vi "Compile Analog Replay 1.0 Data.vi"(7 "RIO Address":string, 8 "error in (no error)":errorcluster, 11 "Device Item Ref in":T3 format="%.0x") -> (0 "error out":errorcluster, 1 "bitfile names":string[](array[string]), 2 "Analog Replays":T1[](array[typedef]), 3 "Device Item Ref out":T3 format="%.0x")   [LabVIEW 2019, in "Engine Simulation Toolkit System Explorer.lvlib"]
uses:
  Engine Simulation Toolkit System Explorer.lvlib
  <vilib>/NI VeriStand/Custom Device API/Custom Device Item Ref.ctl
  Shared/1.0 Analog Replay Engine Data.ctl
  Shared/1.0 Analog Replay FIFO Idxs.ctl
  Position Reference.ctl
  Shared/Properties.vi
  Shared/Constants and GUIDs.vi
  <vilib>/NI VeriStand/Custom Device Tools/Custom Device Utility Library/NI VeriStand - Search for Item by GUID.vi
  <vilib>/NI VeriStand/Custom Device API/Get Item Property (String).vi
  <vilib>/NI VeriStand/Custom Device API/Get Item Property (Boolean).vi
  <vilib>/NI VeriStand/Custom Device API/Get Item Property (U16).vi
  <vilib>/NI VeriStand/Custom Device API/Get Item Property (Double).vi
  Shared/Engine Simulation Toolkit Shared.lvlib
  <vilib>/NI VeriStand/Custom Device API/Custom Device API.lvlib
  <vilib>/NI VeriStand/Custom Device Tools/Custom Device Utility Library/Custom Device Utility Library.lvlib
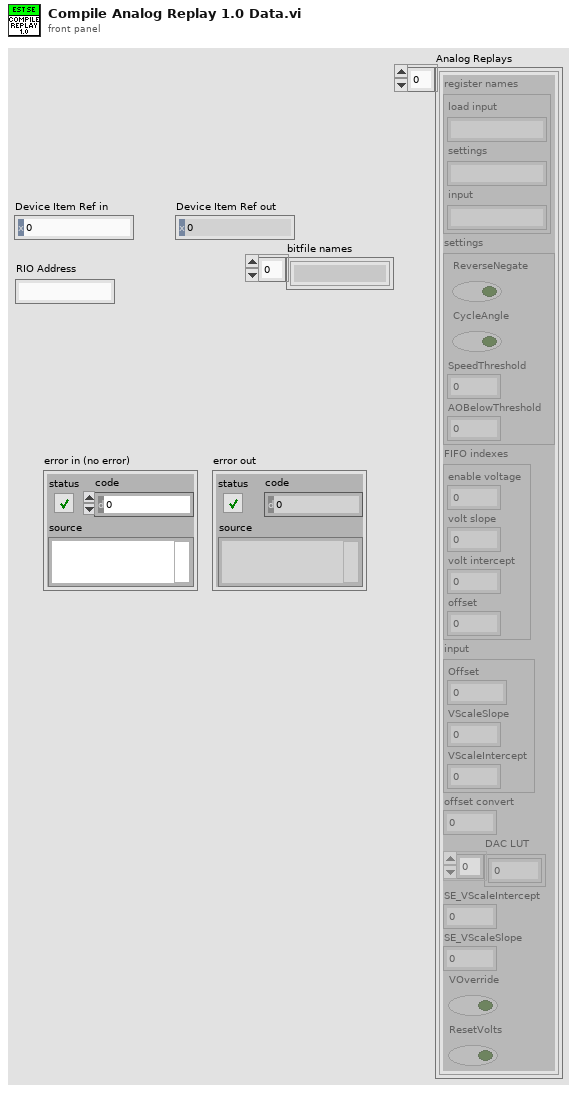
[diagram p1: front panel]
types:
  T1 = typedef "Engine Simulation Toolkit Shared.lvlib/1.0 Analog Replay Engine Data.ctl" = cluster{"register names":cluster{"load input":string, "settings":string, "input":string}, "settings":cluster{"ReverseNegate":bool, "CycleAngle":bool, "SpeedThreshold":fxp<+/-,23,2>, "AOBelowThreshold":i16}, "FIFO indexes":T2, "input":cluster{"Offset":i16, "VScaleSlope":fxp<+,18,6>, "VScaleIntercept":fxp<+/-,18,3>}, "offset convert":dbl, "DAC LUT":i16[], "SE_VScaleIntercept":fxp<+/-,18,3>, "SE_VScaleSlope":fxp<+,18,6>, "VOverride":bool, "ResetVolts":bool}
  T2 = typedef "Engine Simulation Toolkit Shared.lvlib/1.0 Analog Replay FIFO Idxs.ctl" = cluster{"enable voltage":i32, "volt slope":i32, "volt intercept":i32, "offset":i32}
  T3 = typedef "Custom Device API.lvlib/Custom Device Item Ref.ctl" = u64
  T4 = typedef "Engine Simulation Toolkit System Explorer.lvlib/Position Reference.ctl" = enum16{"Crank angle", "Cycle angle"}
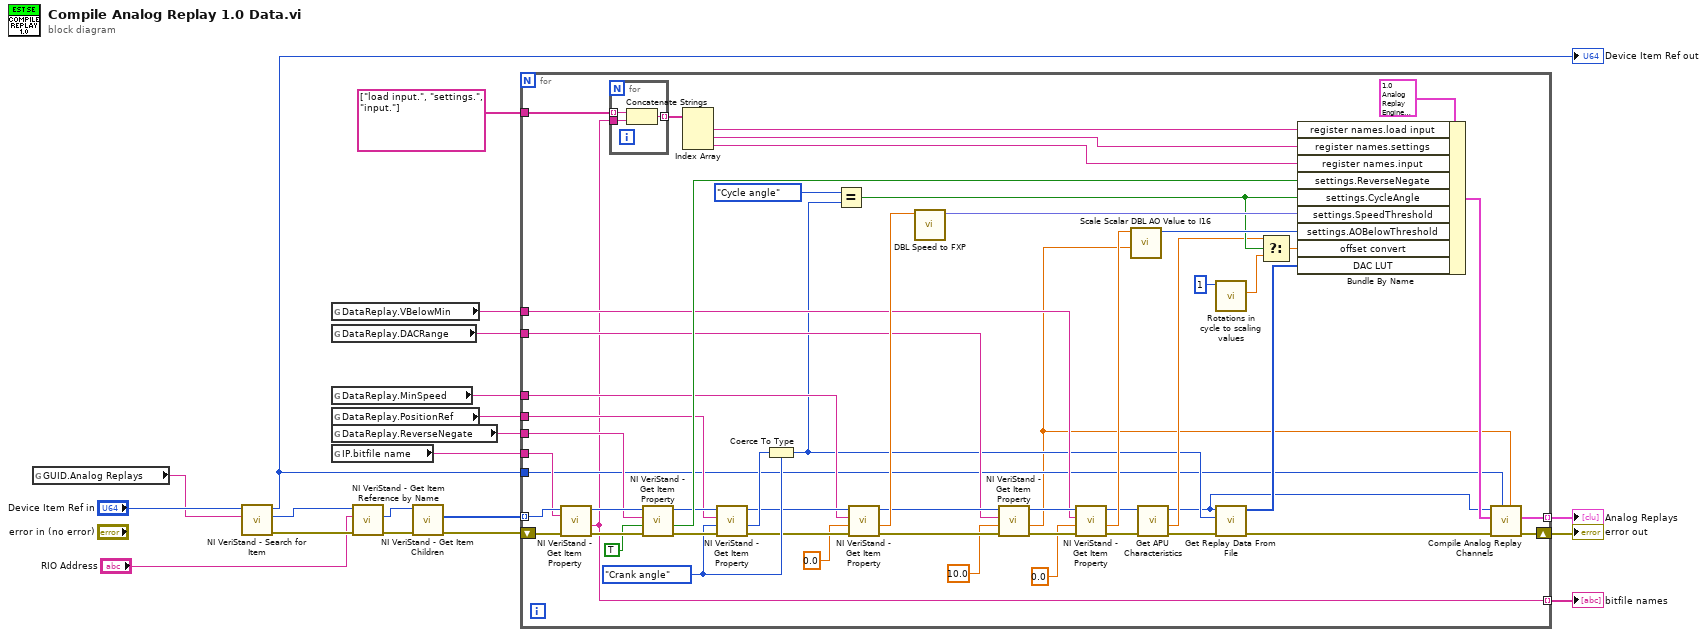
[diagram p0: block diagram]
diagram:
  n1 = global read "Constants and GUIDs.vi" "GUID.Analog Replays"() -> (w7:string)
  n2 = call-poly <vilib>:"NI VeriStand - Search for Item.vi"("Item GUID"=w7, "Section Ref in"="Device Item Ref in") -> ("error out"=w3:errorcluster, "Item Ref"=w6:T3, "Section Ref out"=w1:T3)  [unwired: 6 in, 1 out]
  "Device Item Ref out" <- w1
  n3 = global read "Properties.vi" "DataReplay.VBelowMin"() -> (w11:string)
  n4 = global read "Properties.vi" "DataReplay.DACRange"() -> (w12:string)
  n5 = global read "Properties.vi" "DataReplay.MinSpeed"() -> (w14:string)
  n6 = global read "Properties.vi" "DataReplay.PositionRef"() -> (w15:string)
  n7 = global read "Properties.vi" "DataReplay.ReverseNegate"() -> (w17:string)
  n8 = global read "Properties.vi" "IP.bitfile name"() -> (w19:string)
  n9 = call <vilib>:"NI VeriStand - Get Item Reference by Name.vi"("error in (no error)"=w3, "Item Name"="RIO Address", "Parent Ref in"=w6) -> ("error out"=w4:errorcluster, "Item Ref"=w5:T3)  [unwired: 5 in, 2 out]
  n10 = call <vilib>:"NI VeriStand - Get Item Children.vi"("error in (no error)"=w4, "Item Ref in"=w5) -> ("error out"=w20:errorcluster, "Child Refs"=w13:T3[])  [unwired: 6 in, 2 out]
  n11 = for {
    shift-right: [w29] -> w16
    shift-left: w20 -> [w74]
    tunnel: w13 -> [w73] mode=indexing
    tunnel: w19 -> [w72]
    tunnel: string[] ["load input.", "settings.", "input."] -> [w71]
    tunnel: w17 -> [w64]
    tunnel: w15 -> [w59]
    tunnel: w14 -> [w52]
    tunnel: w1 -> [w24]
    tunnel: w12 -> [w46]
    tunnel: w11 -> [w42]
    tunnel: [w26] -> w10 mode=indexing
    tunnel: [w21] -> w9 mode=indexing
    w58 = Position_Reference."Crank angle" ("Position reference")
    n12 = call-poly <vilib>:"NI VeriStand - Get Item Property.vi"("error in (no error)"=w74, "Property Name"=w72, "Item Ref in"=w73) -> ("error out"=w65:errorcluster, "Value"=w21:string, "Item Ref out"=w66:T3)  [unwired: 5 in, 1 out]
    n13 = for {
      tunnel: w21 -> [w77]
      tunnel: w71 -> [w76] mode=indexing
      tunnel: [w75] -> w69 mode=indexing
      n14 = Concatenate Strings(w76, w77) -> (w75:string)
    }
    n15 = call-poly <vilib>:"NI VeriStand - Get Item Property.vi"("error in (no error)"=w65, "Default Value"=TRUE, "Property Name"=w64, "Item Ref in"=w66) -> ("error out"=w60:errorcluster, "Value"=w63:bool, "Item Ref out"=w61:T3)  [unwired: 4 in, 1 out]
    n16 = Index Array(array=w69) -> (element #1=w68:string, element #2=w67:string, element #3=w23:string)  [unwired: 3 in]
    n17 = call-poly <vilib>:"NI VeriStand - Get Item Property.vi"("error in (no error)"=w60, "Default Value"=w58, "Property Name"=w59, "Item Ref in"=w61) -> ("error out"=w55:errorcluster, "Value"=w57:u16, "Item Ref out"=w53:T3)  [unwired: 4 in, 1 out]
    n18 = Coerce To Type(0:w57, 1:w58) -> (2:w32:T4)
    n19 = Equal?(x=Position_Reference."Cycle angle" ("Position reference"), y=w32) -> (x = y?=w37:bool)
    n20 = call-poly <vilib>:"NI VeriStand - Get Item Property.vi"("error in (no error)"=w55, "Default Value"=0.0, "Property Name"=w52, "Item Ref in"=w53) -> ("error out"=w54:errorcluster, "Value"=w51:dbl, "Item Ref out"=w48:T3)  [unwired: 4 in, 1 out]
    n21 = call "DBL Speed to FXP.vi"("Desired speed (RPM)"=w51) -> ("FXP speed"=w49:fxp<+/-,23,2>)  [unwired: 6 in, 4 out]
    n22 = call-poly <vilib>:"NI VeriStand - Get Item Property.vi"("error in (no error)"=w54, "Default Value"=10.0, "Property Name"=w46, "Item Ref in"=w48) -> ("error out"=w47:errorcluster, "Value"=w22:dbl, "Item Ref out"=w43:T3)  [unwired: 4 in, 1 out]
    n23 = call-poly <vilib>:"NI VeriStand - Get Item Property.vi"("error in (no error)"=w47, "Default Value"=0.0, "Property Name"=w42, "Item Ref in"=w43) -> ("error out"=w44:errorcluster, "Value"=w40:dbl, "Item Ref out"=w38:T3)  [unwired: 4 in, 1 out]
    n24 = call "Scale Scalar DBL AO Value to I16.vi"("DAC bipolar range"=w22, "AO DBL value"=w40) -> ("AO I16 value"=w39:i16)  [unwired: 9 in]
    n25 = call "Get APU Characteristics.vi"("error in (no error)"=w44, "Item Ref in"=w38) -> ("error out"=w31:errorcluster, "angle to u16 scale factor"=w35:dbl, "Item Ref out"=w25:T3)  [unwired: 3 in, 4 out]
    n26 = call "Rotations in cycle to scaling values.vi"("rotations in a cycle"=u16 1) -> ("angle to u16 scale factor"=w34:dbl)  [unwired: 8 in, 2 out]
    n27 = call "Get Replay Data From File.vi"("error in (no error)"=w31, "Position reference"=w32, "Item Ref in"=w25) -> ("error out"=w28:errorcluster, "DAC Data"=w30:i16[])  [unwired: 6 in, 1 out]
    n28 = Select(t=w35, s=w37, f=w34) -> (s? t:f=w33:dbl)
    n29 = Bundle By Name(cluster=T1 {"register names"={"load input"="", "settings"="", "input"=""}, "settings"={"ReverseNegate"=FALSE, "CycleAngle"=FALSE, "SpeedThreshold"=0.0, "AOBelowThreshold"=0}, "FIFO indexes"={"enable voltage"=0, "volt slope"=0, "volt intercept"=0, "offset"=0}, "input"={"Offset"=0, "VScaleSlope"=0.0, "VScaleIntercept"=0.0}, "offset convert"=0.0, "DAC LUT"=[], "SE_VScaleIntercept"=0.0, "SE_VScaleSlope"=0.0, "VOverride"=FALSE, "ResetVolts"=FALSE} ("1.0.0 Analog Replay"), "register names.load input"=w68, "register names.settings"=w67, "register names.input"=w23, "settings.ReverseNegate"=w63, "settings.CycleAngle"=w37, "settings.SpeedThreshold"=w49, "settings.AOBelowThreshold"=w39, "offset convert"=w33, "DAC LUT"=w30) -> (w27:T1)
    n30 = call "Compile Analog Replay Channels.vi"("DAC bipolar range"=w22, "Custom device ref"=w24, "error in (no error)"=w28, "1.0.0 Analog Replay in"=w27, "Item Ref in"=w25) -> ("error out"=w29:errorcluster, "1.0.0 Analog Replay out"=w26:T1)  [unwired: 5 in]
  }
  "error out" <- w16
  "Analog Replays" <- w10
  "bitfile names" <- w9
